vi "Divide Polynomials.vi"   [LabVIEW 2020, in "NI_AALPro.lvlib"]
doc: "Divides polynomial <B>P(x)</B> by polynomial <B>Q(x)</B>. The data types you wire to the <B>P(x)</B> and <B>Q(x)</B> inputs determine the polymorphic instance to use."
uses:
  NI_AALPro.lvlib
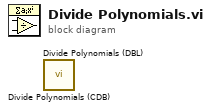
[diagram p0: block diagram]
diagram:
  n1 = call "Divide Polynomials (CDB).vi"() -> ()  [unwired: 9 in, 3 out]
  n2 = call "Divide Polynomials (DBL).vi"() -> ()  [unwired: 9 in, 3 out]
